vi "Table to report table.vi"() -> ()   [LabVIEW 2021]
panel:
  out "appended array":string[][](array[string])
  in  "Array":string[](array[string])
  in  "tdms file":refnum<k34>
  out "tdms file out":refnum<k34>
  out "column Header Strings[]":string[](array[string])
  out "NaN/Path/Refnum?":bool[][](array[boolean])
  in  "group name in":string
  out "Table out":string[][](array[string])=[["3", "3", "3"], ["k", "k", "l"], ["l", "k", "k"], ["k", "k", ""], ["k", "", ""]]
  in  "Table in":string[][](table)
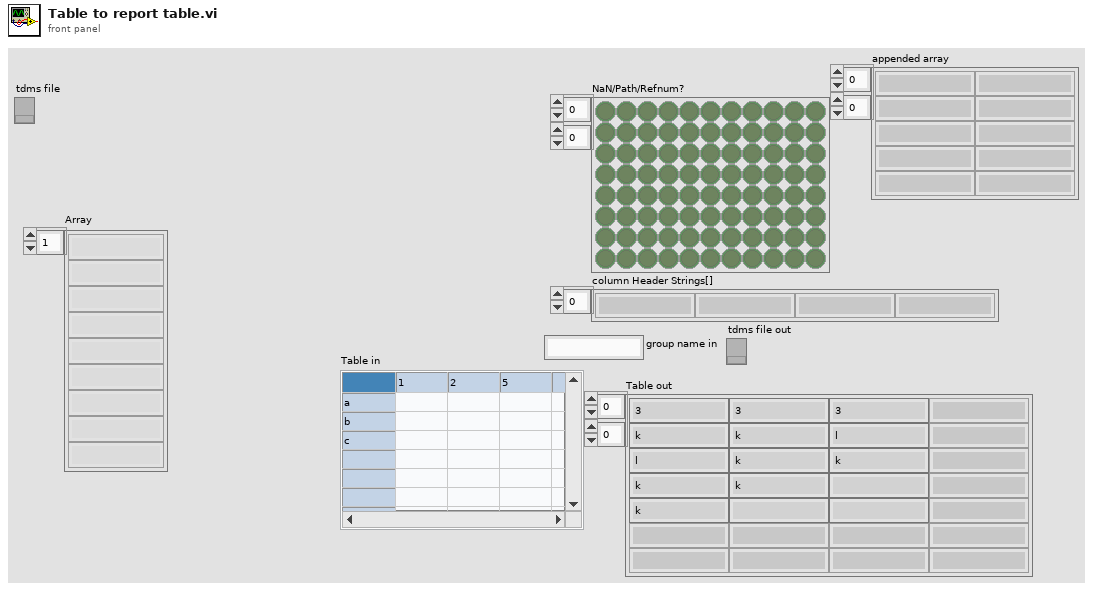
[diagram p1: front panel]
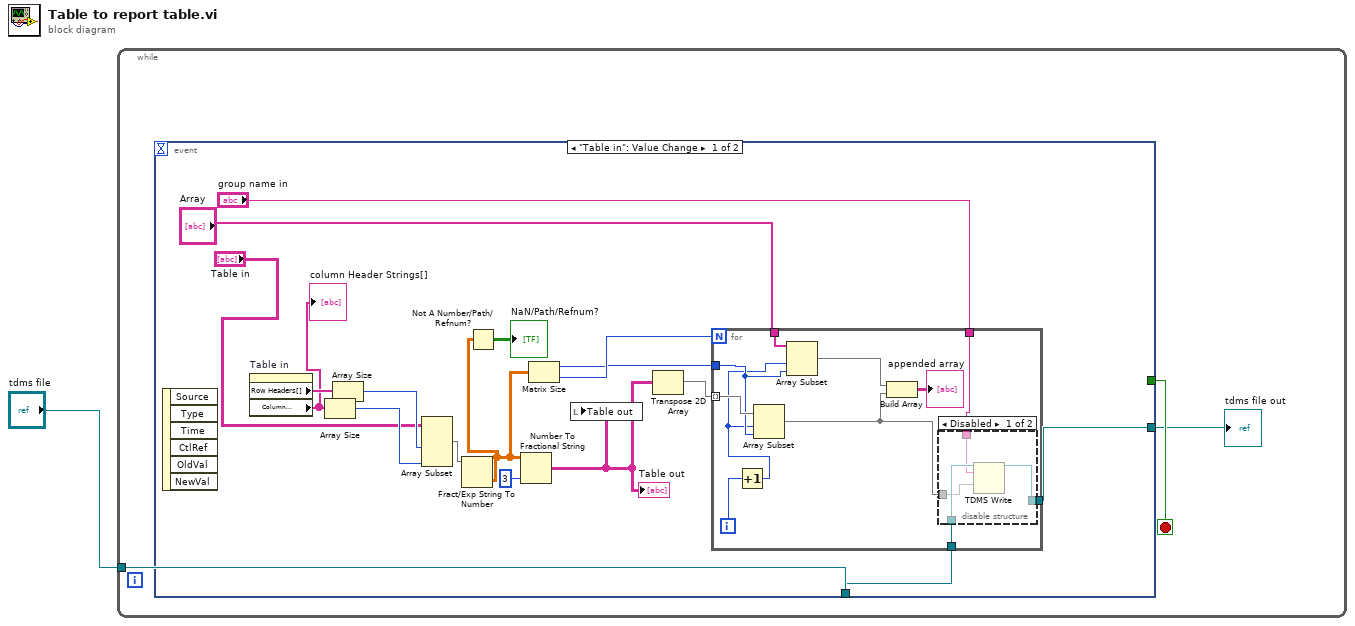
[diagram p0: block diagram]
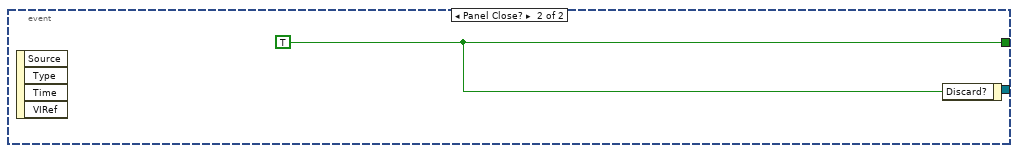
[diagram p3: hidden frame]
diagram:
  n1 = while {
    tunnel: "tdms file" -> [w2]
    stop <- w4 stop-if-true
    n2 = event shown="[0] \"Table in\": Value Change" {
      selector: _ -> [_ _]
      dyn-events: _ -> [_ _]
      timeout: _ -> [_ _]
      tunnel: [_ w37] -> w4
      tunnel: [w6 _] -> w3
      tunnel: w2 -> [w8 _]
      event "Table in": Value Change {
        n3 = event-data() -> ()  [unwired: 1 in, 6 out]
        n4 = property on="Table in" class="Tbl (strict)"() -> ("Row Headers[]"=w21:string[], "Column Headers[]"=w10:string[])  [unwired: 2 in, 2 out]
        "column Header Strings[]" <- w10
        n5 = Array Size(array=w10) -> (size(s)=w20:i32)
        n6 = Array Size(array=w21) -> (size(s)=w19:i32)
        n7 = Array Subset(array="Table in", length (row)=w19, length (col)=w20) -> (w18:string[][])  [unwired: 2 in]
        n8 = Fract/Exp String To Number(string=w18) -> (number=w13:dbl[][])  [unwired: 3 in, 1 out]
        n9 = Not A Number/Path/Refnum?(number/path/refnum=w13) -> (NaN/Path/Refnum?=→"NaN/Path/Refnum?":bool[][])
        n10 = Number To Fractional String(number=w13, precision (6)=i16 3) -> (F-format string=w14:string[][])  [unwired: 2 in]
        "Table out" <- w14
        n11 = Matrix Size(0:w13) -> (1:w5:i32, 2:w16:i32)
        n12 = local write "Table out"(w14) -> ()
        n13 = Transpose 2D Array(2D array=w14) -> (transposed array=w15:string[][])
        n14 = for {
          N: w16 -> [_]
          tunnel: w15 -> [w32] mode=indexing
          tunnel: "Array" -> [w31]
          tunnel: w8 -> [w27]
          tunnel: "group name in" -> [w26]
          tunnel: [w25] -> w6
          tunnel: w5 -> [w24]
          i -> [w23]
          n15 = Increment(x=w23) -> (x+1=w22:i32)
          n16 = Array Subset(array=w32, index=w22, length=w24) -> (w29:string[])
          n17 = Array Subset(array=w31, index=w22, length=w24) -> (w30:string[])
          n18 = Build Array(w30, w29) -> (→"appended array":string[][])
          n19 = disable-structure shown="Disabled" {
            disable-tunnel: w27 -> [w36 _]
            disable-tunnel: w26 -> [w35 _]
            disable-tunnel: w29 -> [w34 _]
            disable-tunnel: [w33 _] -> w25
            frame Disabled {
              n20 = TDMS Write(0:w36, 5:w35, 9:w34) -> (4:w33:refnum<k34>)  [unwired: 3 in, 3 out]
            }
            frame Enabled {
            }
          }
        }
      }
      event Panel Close? {
        w37 = TRUE ("Discard?")
        n21 = event-data() -> ()  [unwired: 1 in, 4 out]
        n22 = event-data("Discard?"=w37) -> ()  [unwired: 1 in, 1 out]
      }
    }
    "tdms file out" <- w3
  }
